vi "Max Bits Left.vi"(8 "error in (no error)":errorcluster, 11 "Packet in":refnum<class "Packet.lvclass">) -> (0 "error out":errorcluster, 2 "Max Bits Left":i32, 3 "Packet out":refnum<class "Packet.lvclass">)   [LabVIEW 2020, in "Packet.lvclass"]
uses:
  Packet.lvclass
  Packet.lvclass/Packet.ctl
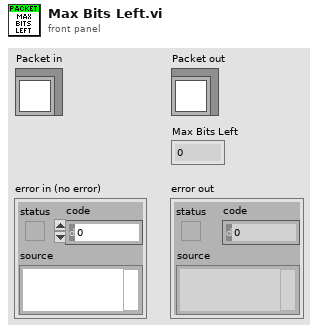
[diagram p1: front panel]
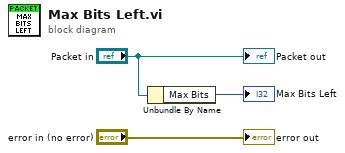
[diagram p0: block diagram]
diagram:
  n1 = Unbundle By Name("Packet in") -> ("Max Bits"=→"Max Bits Left":i32)
  "error out" <- "error in (no error)"
  "Packet out" <- "Packet in"
